vi "2017-01-20 2DScanAndHold.vi"() -> ()   [LabVIEW 2016]
uses:
  <vilib>/Utility/error.llb/DialogType.ctl
  <vilib>/DAQmx/write.llb/DAQmx Write (Analog 1D DBL NChan 1Samp).vi
  <vilib>/DAQmx/write.llb/DAQmx Write (Analog DBL 1Chan 1Samp).vi
  <vilib>/DAQmx/create/channels.llb/DAQmx Create Channel (AO-Voltage-Basic).vi
  <vilib>/DAQmx/miscellaneous.llb/DAQmx Fill In Error Info.vi
panel:
  in  "Mode":enum32{"Hold", "Scan"}(radio)
  in  "Max Voltage 3":dbl=10.0
  in  "Min Voltage Voltage 2":dbl=-10.0
  in  "Physical Channel(s)":tag="Dev1/ao0"
  out "Current Voltage 2":dbl
  out "Next Voltage 2":dbl
  in  "Wait Time (ms) 2":dbl=100.0
  in  "Voltage Step 2":dbl=0.1
  in  "Physical Channel(s)":tag="Dev1/ao0"
  in  "Stop 2":bool
  in  "Output Voltage 2":dbl[](array[numeric])
  in  "Min Voltage 2":dbl=-10.0
  in  "Max Voltage 2":dbl=10.0
  in  "Min Voltage":dbl=-10.0
  in  "Max Voltage":dbl=10.0
  in  "Output Voltage":dbl[](array[numeric])
  in  "Wait Time (ms)":dbl=100.0
  in  "Mode":enum32{"Hold", "Scan"}(radio)
  in  "Stop":bool
  in  "Physical Channel(s)":tag="Dev1/ao0"
  out "Next Voltage":dbl
  out "Current Voltage":dbl
  in  "Voltage Step":dbl=0.1
  in  "Physical Channel(s)":tag="Dev1/ao0"
  in  "Min Voltage Voltage":dbl=-10.0
  in  "Max Voltage":dbl=10.0
  # "Hold"
  # "Scan"
  # "USE THIS STOP BUTTON (FOR NOW)"
  # "Y Control:\nMake sure both physical channels set to ao0"
  # "X Control:\nMake sure both physical channels set to ao1"
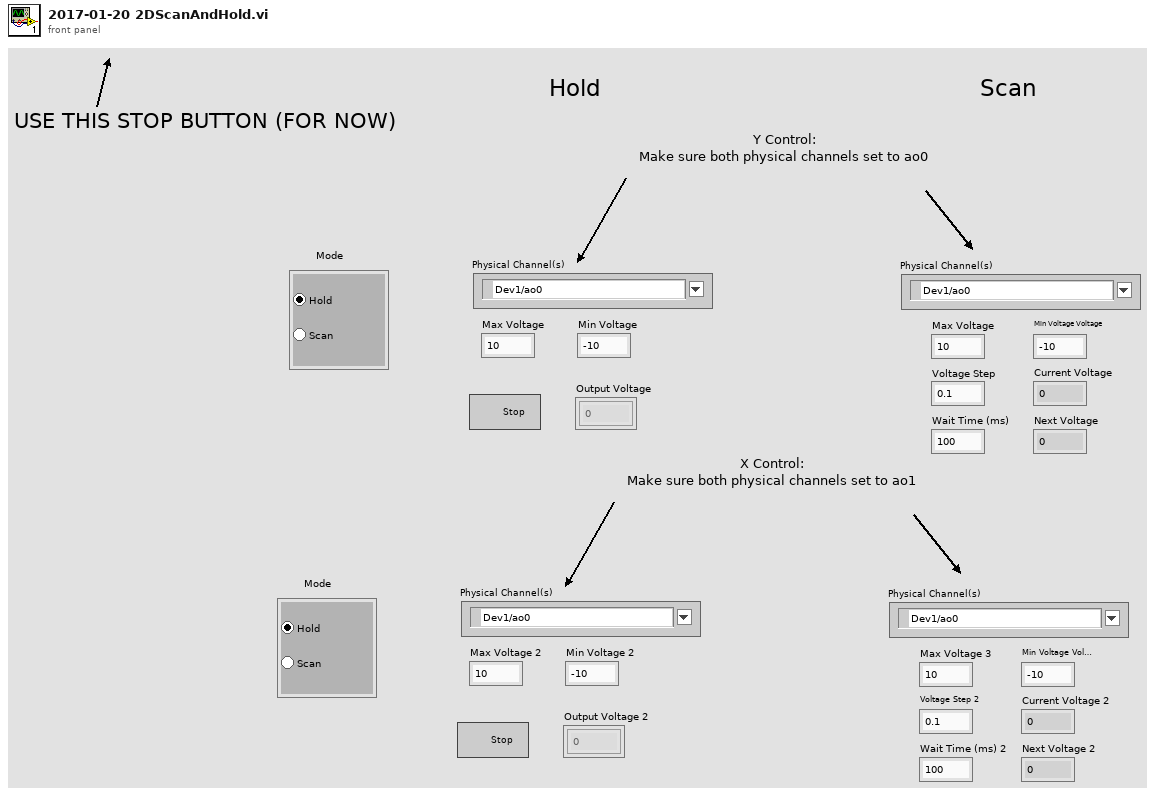
[diagram p1: front panel]
types:
  T1 = typedef "DialogType.ctl" = u16
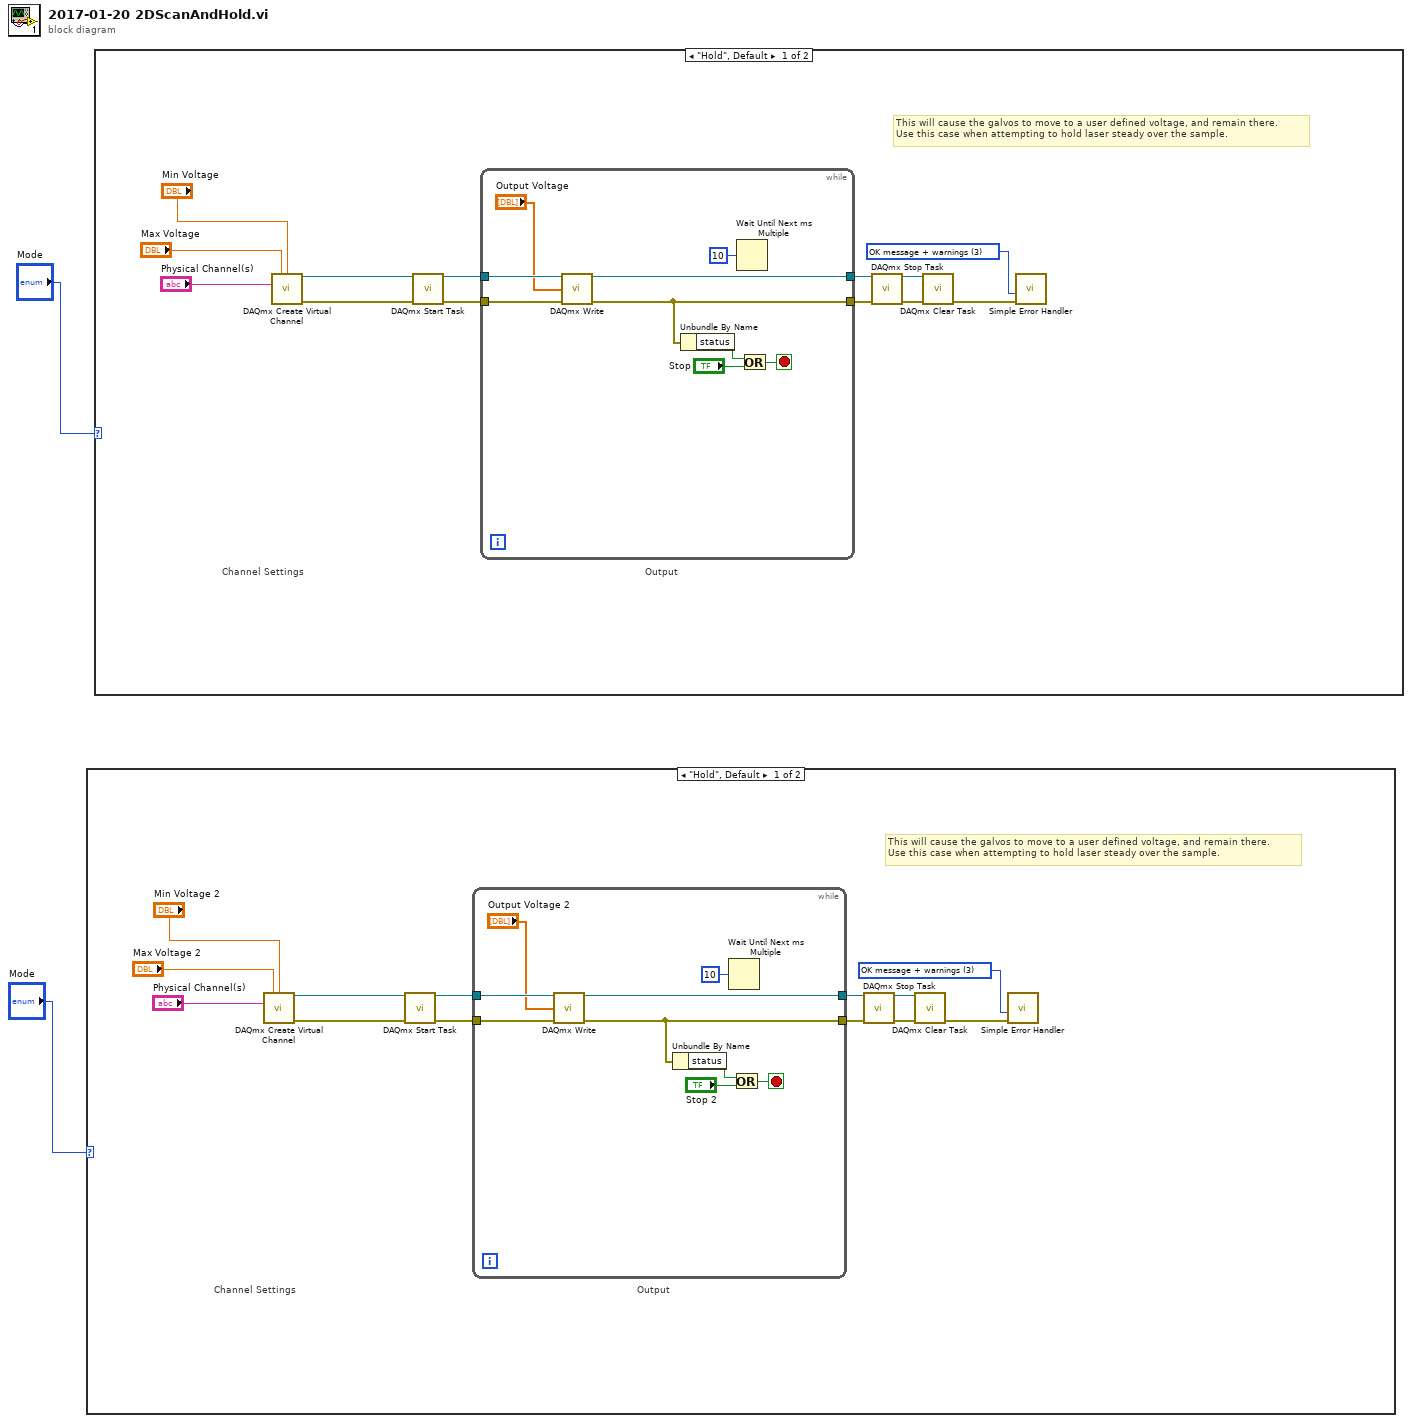
[diagram p0: block diagram]
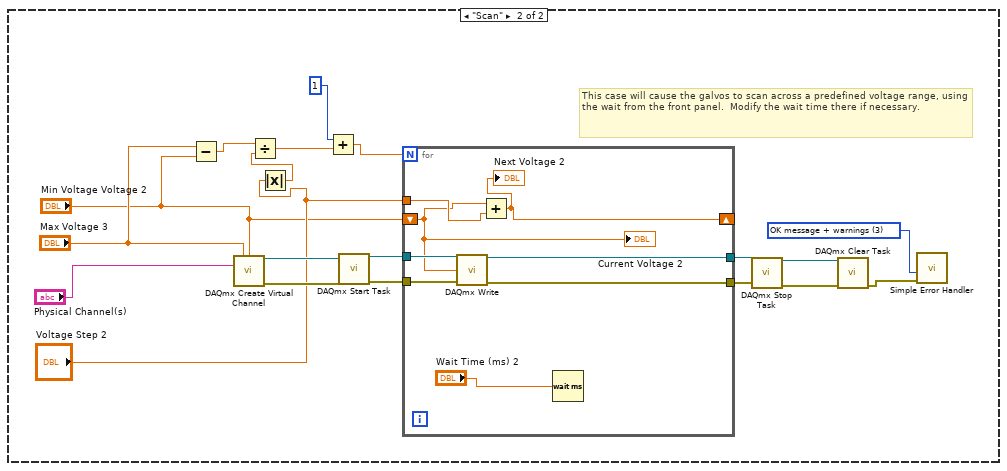
[diagram p2: hidden frame]
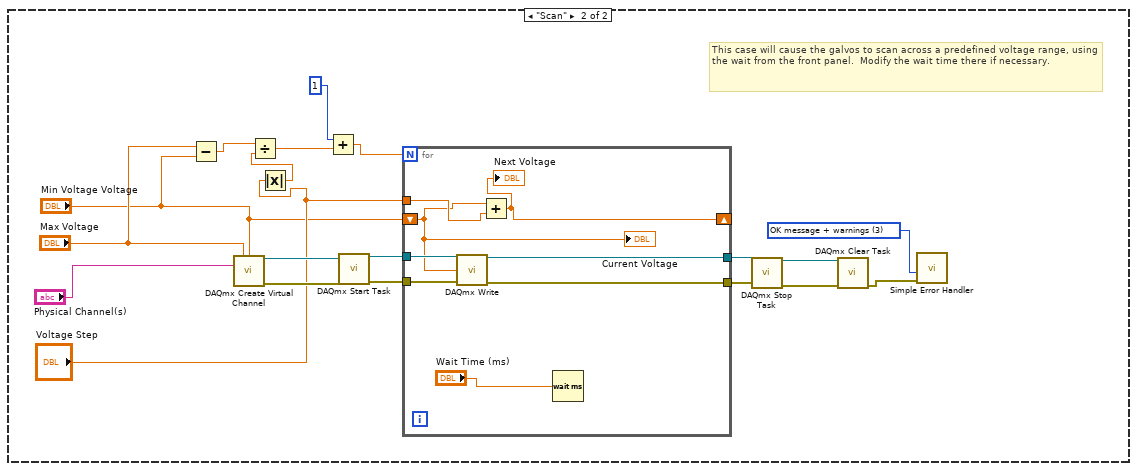
[diagram p3: hidden frame]
diagram:
  n1 = case shown="\"Hold\", Default" "Mode" {
    frame "Hold", Default {
      w5 = T1 3 items=["no dialog", "OK message", "continue or stop message", "OK message + warnings", "continue/stop + warnings"] ("type of dialog (OK msg:1)")
      # "This will cause the galvos to move to a user defined voltage, and remain there.\nUse this case when attempting to hold laser steady over the sample."
      # "Output"
      # "Channel Settings"
      n2 = call-poly <vilib>:"DAQmx Create Virtual Channel.vi"("maximum value"="Max Voltage 2", "minimum value"="Min Voltage 2", "physical channels"="Physical Channel(s)") -> ("task out"=w13:refnum<k21>, "error out"=w12:errorcluster)  [unwired: 11 in]
      n3 = call <vilib>:"DAQmx Start Task.vi"("task/channels in"=w13, "error in"=w12) -> ("task out"=w11:refnum<k21>, "error out"=w10:errorcluster)  [unwired: 12 in]
      n4 = while {
        tunnel: w11 -> [w24]
        tunnel: w10 -> [w23]
        tunnel: [w18] -> w8
        tunnel: [w22] -> w9
        stop <- w16 stop-if-true
        n5 = call-poly <vilib>:"DAQmx Write.vi"("task/channels in"=w24, "data"="Output Voltage 2", "error in"=w23) -> ("task out"=w22:refnum<k21>, "error out"=w18:errorcluster)  [unwired: 10 in, 1 out]
        n6 = Unbundle By Name(w18) -> ("status"=w20:bool)
        n7 = Wait Until Next ms Multiple(millisecond multiple=u32 10) -> ()  [unwired: 1 out]
        n8 = Or(x=w20, y="Stop 2") -> (x .or. y?=w16:bool)
      }
      n9 = call <vilib>:"DAQmx Stop Task.vi"("task/channels in"=w9, "error in"=w8) -> ("task out"=w7:refnum<k21>, "error out"=w6:errorcluster)  [unwired: 12 in]
      n10 = call <vilib>:"DAQmx Clear Task.vi"("task in"=w7, "error in"=w6) -> ("error out"=w15:errorcluster)  [unwired: 13 in]
      n11 = call <vilib>:"Simple Error Handler.vi"("type of dialog (OK msg:1)"=w5, "error in (no error)"=w15) -> ()  [unwired: 3 in, 5 out]
    }
    frame "Scan" {
      w34 = T1 3 items=["no dialog", "OK message", "continue or stop message", "OK message + warnings", "continue/stop + warnings"] ("type of dialog (OK msg:1)")
      # "This case will cause the galvos to scan across a predefined voltage range, using the wait from the front panel.  Modify the wait time there if necessary."
      n12 = Subtract(x="Max Voltage 3", y="Min Voltage Voltage 2") -> (x-y=w31:dbl)
      n13 = call-poly <vilib>:"DAQmx Create Virtual Channel.vi"("maximum value"="Max Voltage 3", "minimum value"="Min Voltage Voltage 2", "physical channels"="Physical Channel(s)") -> ("task out"=w42:refnum<k21>, "error out"=w41:errorcluster)  [unwired: 11 in]
      n14 = Absolute Value(x="Voltage Step 2") -> (abs(x)=w29:dbl)
      n15 = Divide(x=w31, y=w29) -> (x/y=w27:dbl)
      n16 = Add(x=1, y=w27) -> (x+y=w25:dbl)
      n17 = call <vilib>:"DAQmx Start Task.vi"("task/channels in"=w42, "error in"=w41) -> ("task out"=w40:refnum<k21>, "error out"=w39:errorcluster)  [unwired: 12 in]
      n18 = for {
        N: w25 -> [_]
        tunnel: w40 -> [w51]
        tunnel: w39 -> [w50]
        tunnel: [w49] -> w38
        tunnel: [w47] -> w37
        tunnel: "Voltage Step 2" -> [w48]
        shift-right: [w45] -> _
        shift-left: "Min Voltage Voltage 2" -> [w46]
        n19 = call-poly <vilib>:"DAQmx Write.vi"("task/channels in"=w51, "data"=w46, "error in"=w50) -> ("task out"=w47:refnum<k21>, "error out"=w49:errorcluster)  [unwired: 10 in, 1 out]
        n20 = Add(x=w46, y=w48) -> (x+y=w45:dbl)
        "Next Voltage 2" <- w45
        n21 = Wait (ms)(milliseconds to wait="Wait Time (ms) 2") -> ()  [unwired: 1 out]
        "Current Voltage 2" <- w46
      }
      n22 = call <vilib>:"DAQmx Stop Task.vi"("task/channels in"=w37, "error in"=w38) -> ("task out"=w35:refnum<k21>, "error out"=w36:errorcluster)  [unwired: 12 in]
      n23 = call <vilib>:"DAQmx Clear Task.vi"("task in"=w35, "error in"=w36) -> ("error out"=w33:errorcluster)  [unwired: 13 in]
      n24 = call <vilib>:"Simple Error Handler.vi"("type of dialog (OK msg:1)"=w34, "error in (no error)"=w33) -> ()  [unwired: 3 in, 5 out]
    }
  }
  n25 = case shown="\"Hold\", Default" "Mode" {
    frame "Hold", Default {
      w54 = T1 3 items=["no dialog", "OK message", "continue or stop message", "OK message + warnings", "continue/stop + warnings"] ("type of dialog (OK msg:1)")
      # "This will cause the galvos to move to a user defined voltage, and remain there.\nUse this case when attempting to hold laser steady over the sample."
      # "Output"
      # "Channel Settings"
      n26 = call-poly <vilib>:"DAQmx Create Virtual Channel.vi"("maximum value"="Max Voltage", "minimum value"="Min Voltage", "physical channels"="Physical Channel(s)") -> ("task out"=w62:refnum<k21>, "error out"=w61:errorcluster)  [unwired: 11 in]
      n27 = call <vilib>:"DAQmx Start Task.vi"("task/channels in"=w62, "error in"=w61) -> ("task out"=w60:refnum<k21>, "error out"=w59:errorcluster)  [unwired: 12 in]
      n28 = while {
        tunnel: w60 -> [w73]
        tunnel: w59 -> [w72]
        tunnel: [w67] -> w57
        tunnel: [w71] -> w58
        stop <- w65 stop-if-true
        n29 = call-poly <vilib>:"DAQmx Write.vi"("task/channels in"=w73, "data"="Output Voltage", "error in"=w72) -> ("task out"=w71:refnum<k21>, "error out"=w67:errorcluster)  [unwired: 10 in, 1 out]
        n30 = Unbundle By Name(w67) -> ("status"=w69:bool)
        n31 = Wait Until Next ms Multiple(millisecond multiple=u32 10) -> ()  [unwired: 1 out]
        n32 = Or(x=w69, y="Stop") -> (x .or. y?=w65:bool)
      }
      n33 = call <vilib>:"DAQmx Stop Task.vi"("task/channels in"=w58, "error in"=w57) -> ("task out"=w56:refnum<k21>, "error out"=w55:errorcluster)  [unwired: 12 in]
      n34 = call <vilib>:"DAQmx Clear Task.vi"("task in"=w56, "error in"=w55) -> ("error out"=w64:errorcluster)  [unwired: 13 in]
      n35 = call <vilib>:"Simple Error Handler.vi"("type of dialog (OK msg:1)"=w54, "error in (no error)"=w64) -> ()  [unwired: 3 in, 5 out]
    }
    frame "Scan" {
      w83 = T1 3 items=["no dialog", "OK message", "continue or stop message", "OK message + warnings", "continue/stop + warnings"] ("type of dialog (OK msg:1)")
      # "This case will cause the galvos to scan across a predefined voltage range, using the wait from the front panel.  Modify the wait time there if necessary."
      n36 = Subtract(x="Max Voltage", y="Min Voltage Voltage") -> (x-y=w80:dbl)
      n37 = call-poly <vilib>:"DAQmx Create Virtual Channel.vi"("maximum value"="Max Voltage", "minimum value"="Min Voltage Voltage", "physical channels"="Physical Channel(s)") -> ("task out"=w91:refnum<k21>, "error out"=w90:errorcluster)  [unwired: 11 in]
      n38 = Absolute Value(x="Voltage Step") -> (abs(x)=w78:dbl)
      n39 = Divide(x=w80, y=w78) -> (x/y=w76:dbl)
      n40 = Add(x=1, y=w76) -> (x+y=w74:dbl)
      n41 = call <vilib>:"DAQmx Start Task.vi"("task/channels in"=w91, "error in"=w90) -> ("task out"=w89:refnum<k21>, "error out"=w88:errorcluster)  [unwired: 12 in]
      n42 = for {
        N: w74 -> [_]
        tunnel: w89 -> [w100]
        tunnel: w88 -> [w99]
        tunnel: [w98] -> w87
        tunnel: [w96] -> w86
        tunnel: "Voltage Step" -> [w97]
        shift-right: [w94] -> _
        shift-left: "Min Voltage Voltage" -> [w95]
        n43 = call-poly <vilib>:"DAQmx Write.vi"("task/channels in"=w100, "data"=w95, "error in"=w99) -> ("task out"=w96:refnum<k21>, "error out"=w98:errorcluster)  [unwired: 10 in, 1 out]
        n44 = Add(x=w95, y=w97) -> (x+y=w94:dbl)
        "Next Voltage" <- w94
        n45 = Wait (ms)(milliseconds to wait="Wait Time (ms)") -> ()  [unwired: 1 out]
        "Current Voltage" <- w95
      }
      n46 = call <vilib>:"DAQmx Stop Task.vi"("task/channels in"=w86, "error in"=w87) -> ("task out"=w84:refnum<k21>, "error out"=w85:errorcluster)  [unwired: 12 in]
      n47 = call <vilib>:"DAQmx Clear Task.vi"("task in"=w84, "error in"=w85) -> ("error out"=w82:errorcluster)  [unwired: 13 in]
      n48 = call <vilib>:"Simple Error Handler.vi"("type of dialog (OK msg:1)"=w83, "error in (no error)"=w82) -> ()  [unwired: 3 in, 5 out]
    }
  }
